vi "H5Tis_variable_str.vi"(6 "error in (no error)":errorcluster, 9 "HDF5 Type Ref":T1) -> (0 "error out":errorcluster, 2 "Variable String":bool, 3 "HDF5 Type Ref out":T1)   [LabVIEW 2017]
doc: "Determines whether datatype is a variable-length string."
uses:
  <vilib>/UPVI/lvhdf5/library.llb/HDF5 Ref.ctl
  <vilib>/UPVI/lvhdf5/hdf5.dll
panel:
  # "LVHDF5 Toolkit\nCopyright (c) 2005-2013 by Jason D. Sommerville\nCopyright (c) 2014 by UPVI, LLC.\n\nThis use and distribution of this file is governed by the terms found in \nLICENSE.txt distributed with this toolkit and installed at\n <user.lib>\\_lvhdf5\\LICENSE.txt"
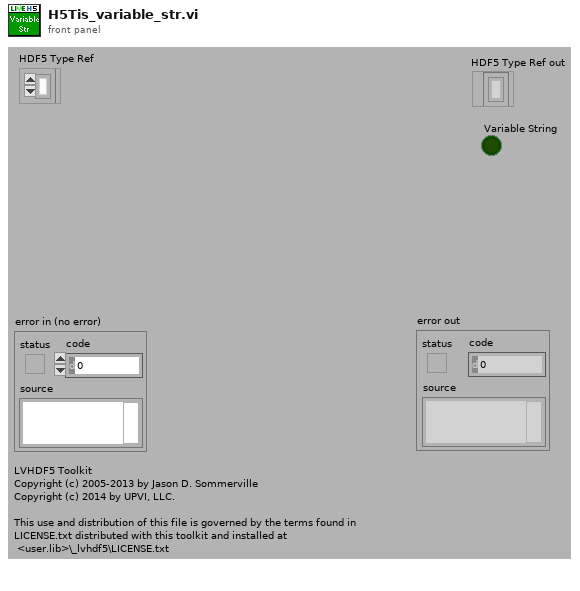
[diagram p1: front panel]
types:
  T1 = typedef "HDF5 Ref.ctl" = refnum<k1>
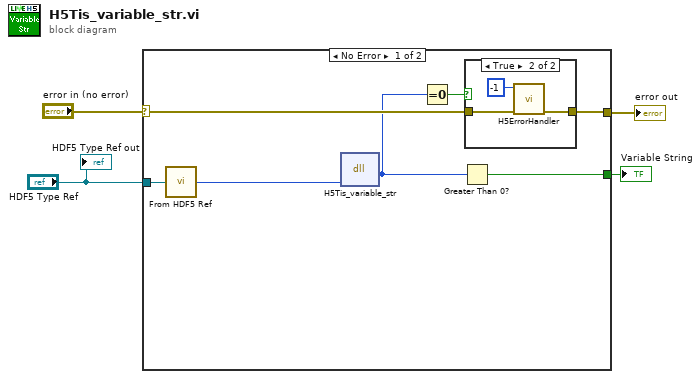
[diagram p0: block diagram]
diagram:
  n1 = case shown="No Error" "error in (no error)" {
    selector: "error in (no error)" -> [w11 w16]
    tunnel: [w10 w16] -> w3
    tunnel: "HDF5 Type Ref" -> [w9 _]
    tunnel: [w5 _] -> w1
    frame No Error {
      n2 = call <vilib>:"From HDF5 Ref.vi"("HDF5 Ref"=w9) -> ("I32"=w8:i32)
      n3 = dll-call lib="C:/Program Files/National Instruments/LabVIEW 2017/vi.lib/UPVI/lvhdf5/hdf5.dll" fn="H5Tis_variable_str"("type_id"=w8) -> (w6:u32)  [unwired: 4 in, 2 out]
      n4 = Equal To 0?(x=w6) -> (x = 0?=w7:bool)
      n5 = Greater Than 0?(x=w6) -> (x > 0?=w5:bool)
      n6 = case shown="True" w7 {
        tunnel: w11 -> [w12 w15]
        tunnel: [w12 w14] -> w10
        frame False {
        }
        frame True {
          n7 = call <vilib>:"H5ErrorHandler.vi"("error in (no error)"=w15, "herr_t"=-1) -> ("error out"=w14:errorcluster)  [unwired: 3 in, 4 out]
        }
      }
    }
    frame Error {
    }
  }
  "error out" <- w3
  "Variable String" <- w1
  "HDF5 Type Ref out" <- "HDF5 Type Ref"
